vi "Botones_intensidad.vi"(2 "Seleción método":bool, 8 "String":string, 9 "Array":dbl[](array[numeric]), 10 "Directorio scripts matlab 2":path=path "C:/Users/franjas/Documents/rutinas-calibracion-slm", 11 "I1":bool) -> (3 "?":bool)   [LabVIEW 2013]
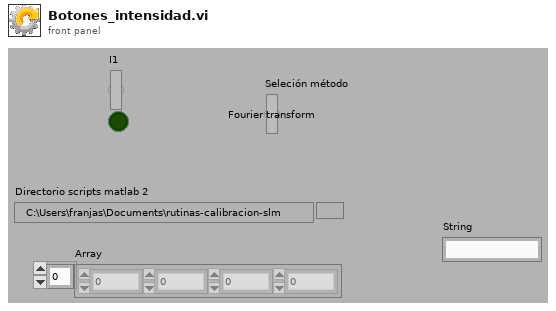
[diagram p1: front panel]
types:
  T1 = enum16{"Escritura", "Med fas", "Conf fase", "Med ampl", "Conf final", "finalizar"}
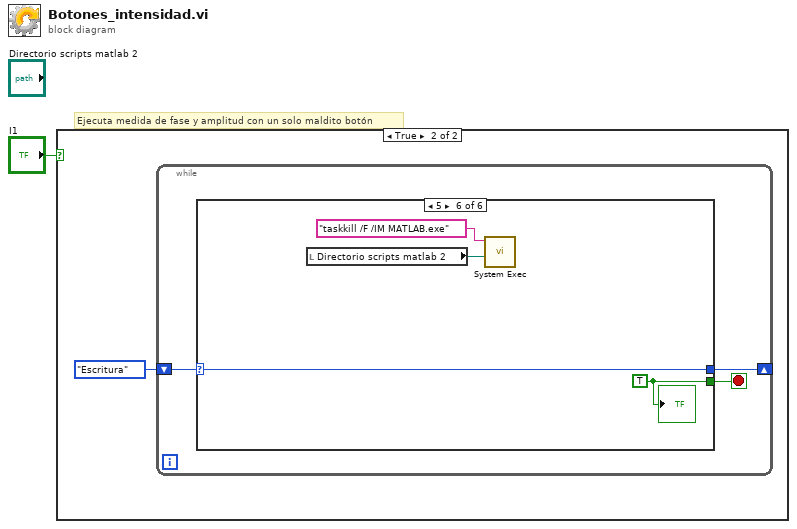
[diagram p0: block diagram]
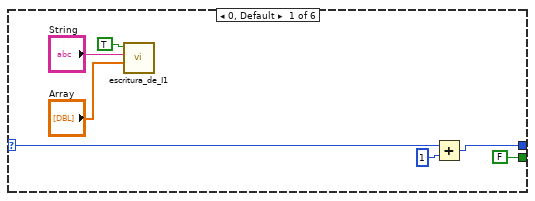
[diagram p3: hidden frame]
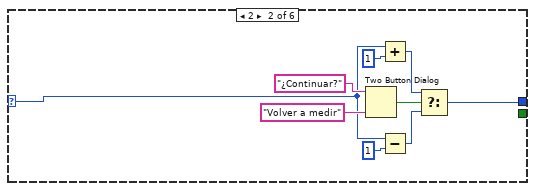
[diagram p4: hidden frame]
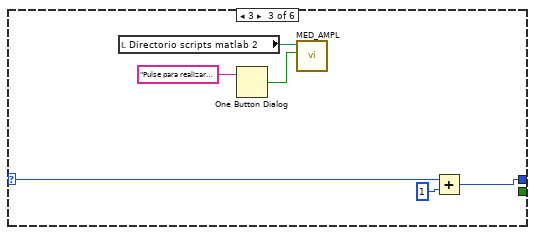
[diagram p5: hidden frame]
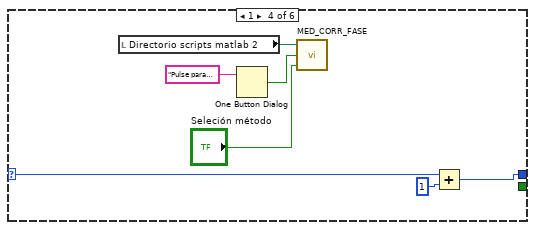
[diagram p6: hidden frame]
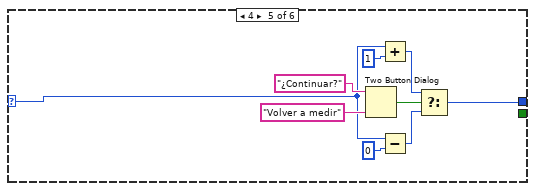
[diagram p7: hidden frame]
diagram:
  # "Ejecuta medida de fase y amplitud con un solo maldito botón"
  n1 = case shown="True" "I1" {
    frame False {
    }
    frame True {
      n2 = while {
        shift-right: [w4] -> _
        shift-left: T1."Escritura" -> [w5]
        stop <- w3 stop-if-true
        n3 = case shown="5" w5 {
          selector: w5 -> [w11 w14 w25 w32 w36 w46]
          tunnel: [w12 w16 w24 w31 w38 w46] -> w4
          tunnel: [FALSE ("I1\n<0,0|0,0>") _ _ _ _ w47] -> w3
          frame 0, Default {
            n4 = call "escritura_de_I1.vi"("I1\n<0,0|0,0>"=TRUE ("I1\n<0,0|0,0>"), "String"="String", "Array"="Array") -> ()  [unwired: 8 in]
            n5 = Add(x=w11, y=1) -> (x+y=w12:i32)
          }
          frame 2 {
            n6 = Two Button Dialog(message="¿Continuar?", 1:"Volver a medir" ("F button name (\"Cancel\")")) -> (T button?=w19:bool)  [unwired: 1 in]
            n7 = Add(x=w14, y=1) -> (x+y=w13:i32)
            n8 = Subtract(x=w14, y=1) -> (x-y=w17:i32)
            n9 = Select(t=w13, s=w19, f=w17) -> (s? t:f=w16:i32)
          }
          frame 3 {
            n10 = local read "Directorio scripts matlab 2"() -> (w22:path)
            n11 = One Button Dialog(message="Pulse para realizar medidas de amplitud:") -> (true=w23:bool)  [unwired: 1 in]
            n12 = call "MED_AMPL.vi"("Boolean"=w23, "Directorio scripts matlab"=w22) -> ()  [unwired: 10 in]
            n13 = Add(x=w25, y=1) -> (x+y=w24:i32)
          }
          frame 1 {
            n14 = local read "Directorio scripts matlab 2"() -> (w29:path)
            n15 = One Button Dialog(message="Pulse para realizar medida de diferencia de fase") -> (true=w30:bool)  [unwired: 1 in]
            n16 = call "MED_CORR_FASE.vi"("Seleción método"="Seleción método", "Ejecucion"=w30, "Directorio scripts matlab"=w29) -> ()
            n17 = Add(x=w32, y=1) -> (x+y=w31:i32)
          }
          frame 4 {
            n18 = Two Button Dialog(message="¿Continuar?", 1:"Volver a medir" ("F button name (\"Cancel\")")) -> (T button?=w41:bool)  [unwired: 1 in]
            n19 = Add(x=w36, y=1) -> (x+y=w35:i32)
            n20 = Subtract(x=w36, y=0) -> (x-y=w39:i32)
            n21 = Select(t=w35, s=w41, f=w39) -> (s? t:f=w38:i32)
          }
          frame 5 {
            w47 = TRUE
            n22 = local read "Directorio scripts matlab 2"() -> (w45:path)
            n23 = call <vilib>:"System Exec.vi"("working directory"=w45, "command line"="taskkill /F /IM MATLAB.exe") -> ()  [unwired: 6 in, 4 out]
            "?" <- w47
          }
        }
      }
    }
  }
